vi "Interpolate 2D Scattered_Create Matrix.vi"(0 "X":dbl[](array[numeric]), 5 "Y":dbl[](array[numeric]), 7 "Z":dbl[](array[numeric])) -> (4 "X(Tri)":dbl[][](array[numeric]), 6 "Y(Tri)":dbl[][](array[numeric]), 8 "Z(Tri)":dbl[][](array[numeric]), 10 "Triangles":i32[][](array[numeric]), 15 "error":i32)   [LabVIEW 2020, in "NI_AAL_Interpolation.lvlib"]
uses:
  <vilib>/gmath/NI_AAL_Interpolation.lvlib
  <vilib>/Analysis/NI_AAL_Geometry.lvlib
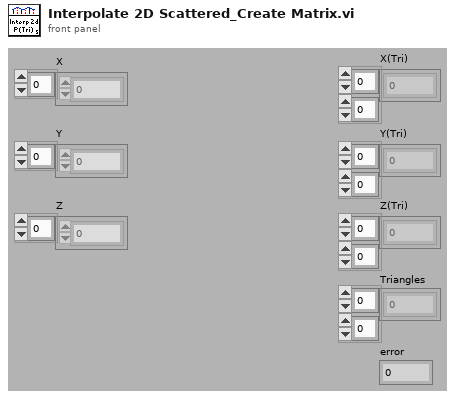
[diagram p1: front panel]
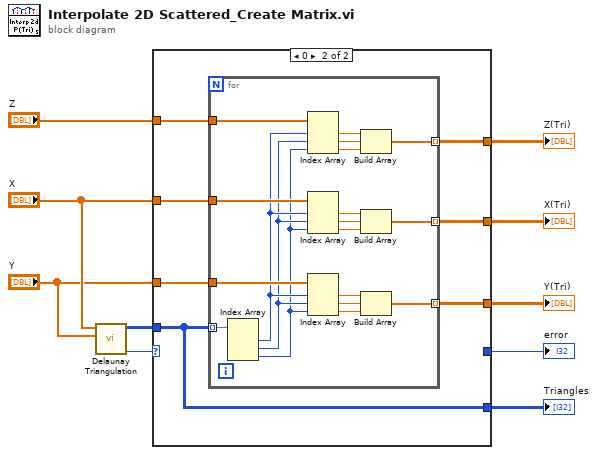
[diagram p0: block diagram]
diagram:
  n1 = call <vilib>:"Delaunay Triangulation.vi"("Y"="Y", "X"="X") -> ("error"=w3:i32, "Triangles"=w10:i32[][])  [unwired: 8 out]
  n2 = case shown="0" w3 {
    selector: w3 -> [w11 _]
    tunnel: w10 -> [_ w12]
    tunnel: "X" -> [_ w18]
    tunnel: "Y" -> [_ w17]
    tunnel: "Z" -> [_ w16]
    tunnel: [_ w15] -> w6
    tunnel: [_ w14] -> w5
    tunnel: [_ w13] -> w4
    tunnel: [_ w12] -> w2
    tunnel: [w11 _] -> w1
    frame -1, Default {
    }
    frame 0 {
      n3 = for {
        tunnel: w12 -> [w34] mode=indexing
        tunnel: w18 -> [w35]
        tunnel: w17 -> [w36]
        tunnel: w16 -> [w37]
        tunnel: [w21] -> w15 mode=indexing
        tunnel: [w20] -> w14 mode=indexing
        tunnel: [w19] -> w13 mode=indexing
        n4 = Index Array(array=w34) -> (element #1=w33:i32, element #2=w32:i32, element #3=w31:i32)  [unwired: 3 in]
        n5 = Index Array(array=w37, index #1=w33, index #2=w32, index #3=w31) -> (element #1=w30:dbl, element #2=w29:dbl, element #3=w28:dbl)
        n6 = Index Array(array=w35, index #1=w33, index #2=w32, index #3=w31) -> (element #1=w24:dbl, element #2=w23:dbl, element #3=w22:dbl)
        n7 = Index Array(array=w36, index #1=w33, index #2=w32, index #3=w31) -> (element #1=w27:dbl, element #2=w26:dbl, element #3=w25:dbl)
        n8 = Build Array(w30, w29, w28) -> (w21:dbl[])
        n9 = Build Array(w24, w23, w22) -> (w20:dbl[])
        n10 = Build Array(w27, w26, w25) -> (w19:dbl[])
      }
    }
  }
  "X(Tri)" <- w5
  "Y(Tri)" <- w4
  "Z(Tri)" <- w6
  "Triangles" <- w2
  "error" <- w1
